vi "Fdx Start (Tx).vi"(6 "Curent Irig Time":T2, 7 "TransmitTime":u32, 8 "error in":errorcluster, 9 "ExtendedStopMode":i32(ring) items=["FDX_ESTOP_NOT_USED", "FDX_ESTOP_EXT_TRG", "FDX_ESTOP_EXT_TRG_RESTART", "FDX_ESTOP_TIME"], 10 "StartMode":i32(ring)=1 items=["FDX_STOP", "FDX_START", "FDX_START_TRG", "FDX_START_TIME"], 11 "InstrumentHandle_port in":u32) -> (0 "error out":errorcluster, 3 "InstrumentHandle_port out":u32)   [LabVIEW 2020, in "AIM664LV.lvlib"]
uses:
  AIM664LV.lvlib
  bsp/AFDX_Controls/IrigTime.ctl
panel:
  in  "TxControl(start)":T1={"StartMode"=1, "Count"=0, "Sign"=0, "Day"=0, "Hour"=0, "Min"=0, "Second"=0, "MilliSec"=0, "MicroSec"=0, "ExtendedStopMode"=0, "TransmitTime"=0} {"StartMode" items=["FDX_STOP", "FDX_START", "FDX_START_TRG", "FDX_START_TIME"]; "ExtendedStopMode" items=["FDX_ESTOP_NOT_USED", "FDX_ESTOP_EXT_TRG", "FDX_ESTOP_EXT_TRG_RESTART", "FDX_ESTOP_TIME"]}
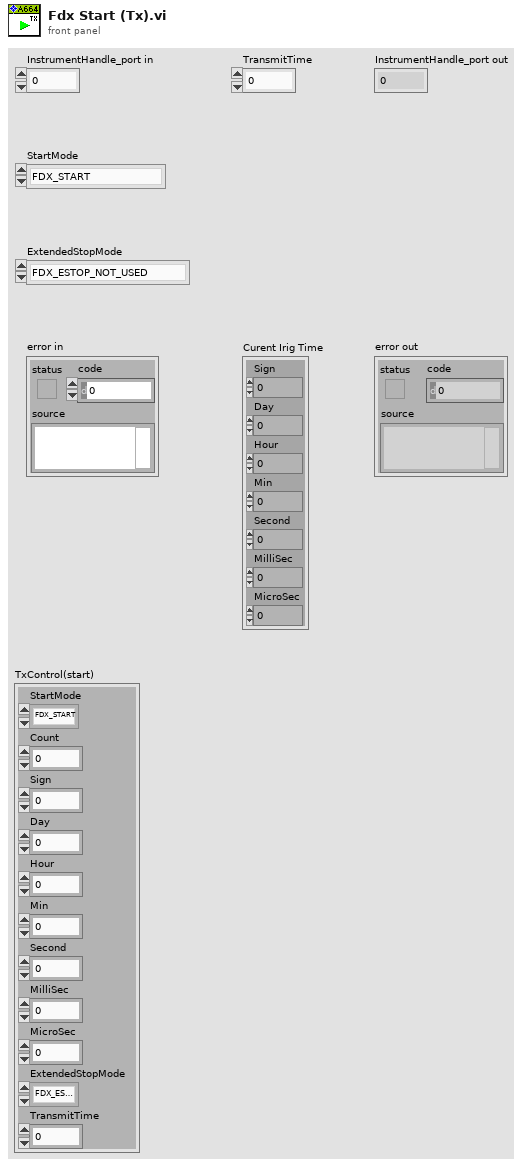
[diagram p1: front panel]
types:
  T1 = cluster{"StartMode":i32, "Count":u32, "Sign":i32, "Day":u32, "Hour":u32, "Min":u32, "Second":u32, "MilliSec":u32, "MicroSec":u32, "ExtendedStopMode":i32, "TransmitTime":u32}
  T2 = typedef "AIM664LV.lvlib/IrigTime.ctl" = cluster{"Sign":i32, "Day":u32, "Hour":u32, "Min":u32, "Second":u32, "MilliSec":u32, "MicroSec":u32}
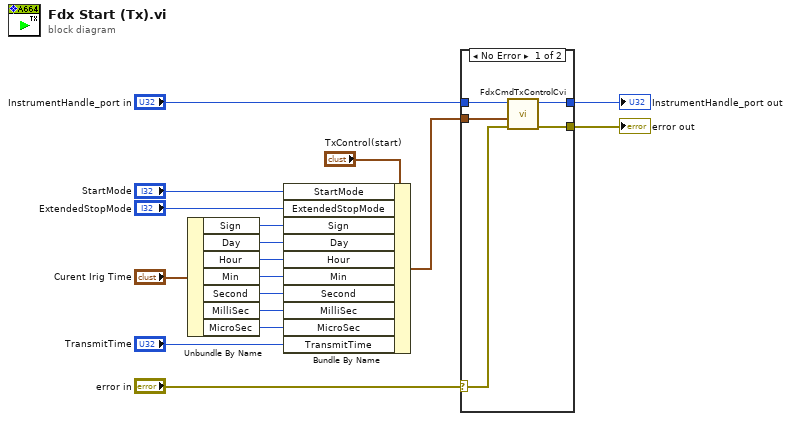
[diagram p0: block diagram]
diagram:
  n1 = Unbundle By Name("Curent Irig Time") -> ("Sign"=w9:i32, "Day"=w8:u32, "Hour"=w7:u32, "Min"=w6:u32, "Second"=w5:u32, "MilliSec"=w4:u32, "MicroSec"=w3:u32)
  n2 = Bundle By Name(cluster="TxControl(start)", "StartMode"="StartMode", "ExtendedStopMode"="ExtendedStopMode", "Sign"=w9, "Day"=w8, "Hour"=w7, "Min"=w6, "Second"=w5, "MilliSec"=w4, "MicroSec"=w3, "TransmitTime"="TransmitTime") -> (w1:T1)
  n3 = case shown="No Error" "error in" {
    selector: "error in" -> [w22 w23]
    tunnel: w1 -> [w21 _]
    tunnel: "InstrumentHandle_port in" -> [w19 w24]
    tunnel: [w20 w23] -> w15
    tunnel: [w18 w24] -> w14
    frame No Error {
      n4 = call "FdxCmdTxControlCvi.vi"("error in"=w22, "TxControl"=w21, "InstrumentHandle_port"=w19) -> ("error out"=w20:errorcluster, "InstrumentHandle_port"=w18:u32)  [unwired: 7 in]
    }
    frame Error {
    }
  }
  "error out" <- w15
  "InstrumentHandle_port out" <- w14
